vi "NF WF1973_74 FM Func.vi"(6 "Read(F)":bool, 7 "Memory No.(1)":i32=1 min=0 max=128 step=1, 8 "error in (no error)":errorcluster caption="Error IN", 9 "Function type(Sin)":u16(ring) items=["Sinusoid", "Square", "Triangle", "Pramp", "Nramp", "Noise", "User"], 10 "Ch(Ch1)":bool, 11 "VISAsession":refnum<visa-resource-name>) -> (0 "error out":errorcluster caption="Error OUT", 2 "Query Function":string, 3 "CopyVISAsession":refnum<visa-resource-name>)   [LabVIEW 2010]
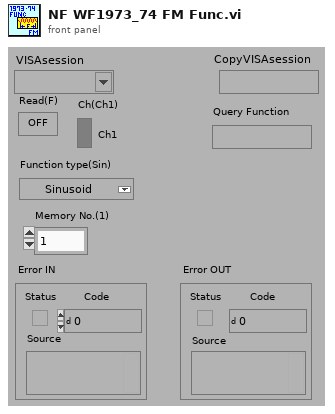
[diagram p1: front panel]
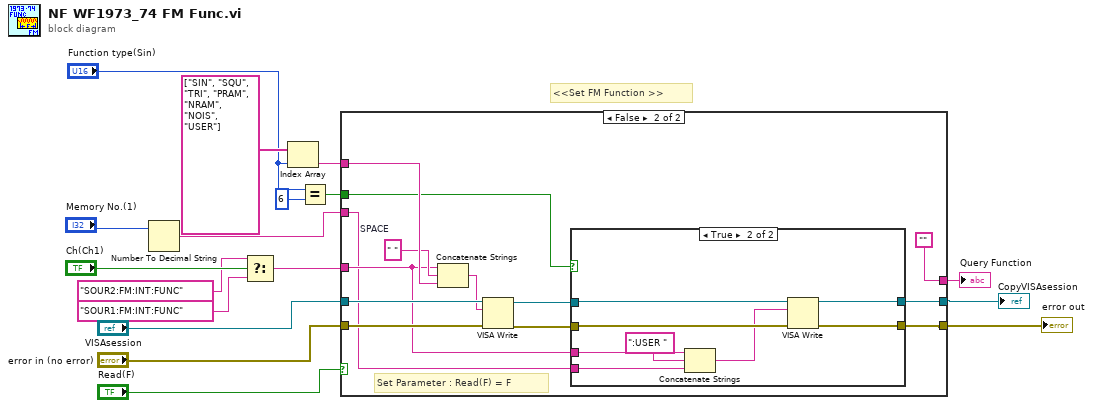
[diagram p0: block diagram]
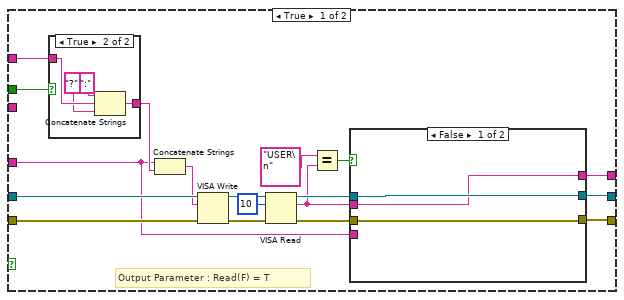
[diagram p2: hidden frame]
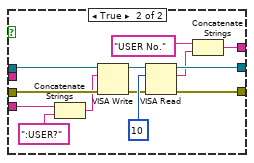
[diagram p3: hidden frame]
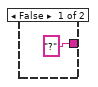
[diagram p4: hidden frame]
diagram:
  # "<<Set FM Function >>"
  n1 = Number To Decimal String(number="Memory No.(1)") -> (decimal integer string=w5:string)  [unwired: 1 in]
  n2 = Select(t="SOUR2:FM:INT:FUNC" ("文字列"), s="Ch(Ch1)", f="SOUR1:FM:INT:FUNC" ("文字列")) -> (s? t:f=w4:string)
  n3 = Index Array(array=string[] ["SIN", "SQU", "TRI", "PRAM", "NRAM", "NOIS", "USER"] ("配列"), index="Function type(Sin)") -> (element=w7:string)
  n4 = Equal?(x="Function type(Sin)", y=u16 6) -> (x = y?=w6:bool)
  n5 = case shown="FALSE" "Read(F)" {
    tunnel: "VISAsession" -> [w35 w69]
    tunnel: [w22 w66] -> w9
    tunnel: [w23 w65] -> w8
    tunnel: "error in (no error)" -> [w32 w68]
    tunnel: w4 -> [w20 w59]
    tunnel: [w21 ""] -> w10
    tunnel: w6 -> [w28 w60]
    tunnel: w5 -> [_ w58]
    tunnel: w7 -> [w29 w62]
    frame True {
      # "Output Parameter : Read(F) = T"
      n6 = case shown="TRUE" w28 {
        tunnel: w29 -> [_ w54]
        tunnel: ["?" ("形式文字列") w56] -> w30
        frame False {
        }
        frame True {
          n7 = Concatenate Strings(":" ("形式文字列"), w54, "?" ("形式文字列")) -> (w56:string)
        }
      }
      n8 = Concatenate Strings(w20, w30) -> (w18:string)
      n9 = VISA Write(VISA resource name=w35, write buffer=w18, error in (no error)=w32) -> (VISA resource name out=w33:refnum<visa-resource-name>, error out=w34:errorcluster)  [unwired: 1 out]
      n10 = VISA Read(VISA resource name=w33, byte count=u32 10 ("バイトカウント（0）"), error in (no error)=w34) -> (VISA resource name out=w25:refnum<visa-resource-name>, read buffer=w19:string, error out=w24:errorcluster)  [unwired: 1 out]
      n11 = Equal?(x="USER\n" ("形式文字列"), y=w19) -> (x = y?=w26:bool)
      n12 = case shown="FALSE" w26 {
        tunnel: w25 -> [w37 w48]
        tunnel: w24 -> [w38 w49]
        tunnel: [w38 w46] -> w23
        tunnel: [w37 w45] -> w22
        tunnel: [w36 w41] -> w21
        tunnel: w20 -> [_ w43]
        tunnel: w19 -> [w36 _]
        frame False {
        }
        frame True {
          n13 = Concatenate Strings(w43, ":USER?" ("形式文字列")) -> (w44:string)
          n14 = VISA Write(VISA resource name=w48, write buffer=w44, error in (no error)=w49) -> (VISA resource name out=w50:refnum<visa-resource-name>, error out=w47:errorcluster)  [unwired: 1 out]
          n15 = VISA Read(VISA resource name=w50, byte count=u32 10 ("バイトカウント（0）"), error in (no error)=w47) -> (VISA resource name out=w45:refnum<visa-resource-name>, read buffer=w39:string, error out=w46:errorcluster)  [unwired: 1 out]
          n16 = Concatenate Strings("USER No." ("形式文字列"), w39) -> (w41:string)
        }
      }
    }
    frame False {
      w61 = " "  # SPACE
      # "Set Parameter : Read(F) = F"
      n17 = Concatenate Strings(w59, w61, w62) -> (w57:string)
      n18 = VISA Write(VISA resource name=w69, write buffer=w57, error in (no error)=w68) -> (VISA resource name out=w64:refnum<visa-resource-name>, error out=w63:errorcluster)  [unwired: 1 out]
      n19 = case shown="TRUE" w60 {
        tunnel: w64 -> [w70 w78]
        tunnel: w63 -> [w71 w79]
        tunnel: [w71 w76] -> w65
        tunnel: [w70 w77] -> w66
        tunnel: w59 -> [_ w74]
        tunnel: w58 -> [_ w72]
        frame False {
        }
        frame True {
          n20 = Concatenate Strings(w74, ":USER " ("文字列"), w72) -> (w75:string)
          n21 = VISA Write(VISA resource name=w78, write buffer=w75, error in (no error)=w79) -> (VISA resource name out=w77:refnum<visa-resource-name>, error out=w76:errorcluster)  [unwired: 1 out]
        }
      }
    }
  }
  "error out" <- w8
  "CopyVISAsession" <- w9
  "Query Function" <- w10
